vi "Test Get Test Name.vi"(8 "error in (no error)":errorcluster, 11 "Test Case In":refnum<class "Test Case Test.lvclass">) -> (0 "error out":errorcluster, 3 "Test Case Out":refnum<class "Test Case Test.lvclass">)   [LabVIEW 2020, in "Test Case Test.lvclass"]
uses:
  Test Case Test.lvclass
  C:/Program Files (x86)/National Instruments/LabVIEW 2020/vi.lib/Astemes/LUnit/Test Case.lvclass
  Test Doubles/Light Test Case Double Copy/Light Test Case Double Copy.lvclass
  C:/git/astemes-lunit/source/Core/LUnit Test Case/LUnit Test Case.lvclass
  source/LUnit Test Case.lvclass/LUnit Test Case.ctl
  <vilib>/Astemes/LUnit/Test Case.lvclass/Test Case.ctl
  e8c5eeff-a694-4c0d-b261-74e2e6f5327d.vi
  <vilib>/Astemes/LUnit/Core/LUnit Test Case/Private/Append Pass Result.vi
  <vilib>/Astemes/LUnit/Core/LUnit Test Case/Private/Append Fail Result.vi
  e8c5eeff-a694-4c0d-b261-74e2e6f5327d.vi/9c5d11cd-9439-4240-a1ee-d9baace9c924.vi
  <vilib>/Astemes/LUnit/Core/LUnit Test Case/Private/Run In UI.vi
  <vilib>/Utility/error.llb/Clear Errors.vi
  <vilib>/Utility/LVClass/Get LV Class Name.vi
  source/LUnit Test Case.lvclass
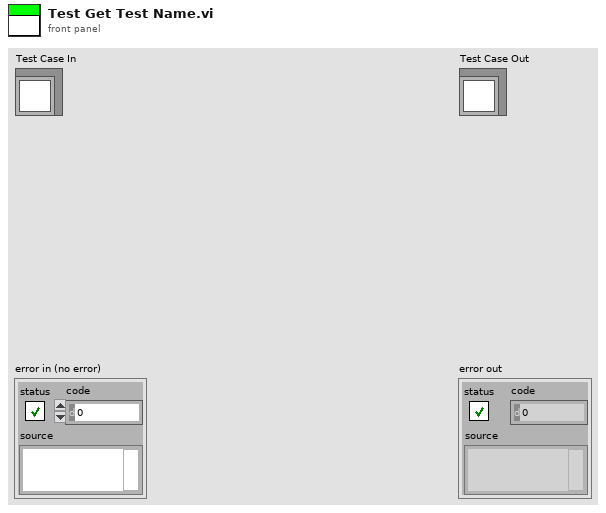
[diagram p1: front panel]
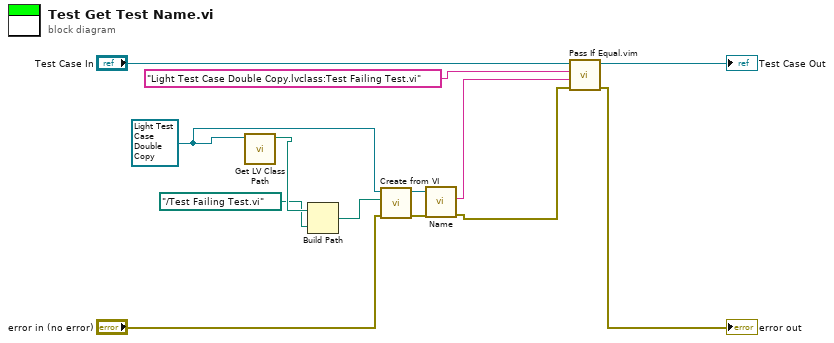
[diagram p0: block diagram]
diagram:
  w2 = refnum<class "Light Test Case Double Copy.lvclass"> refnum ("Light Test Case Double Copy.lvclass")
  n1 = call <vilib>:"Get LV Class Path.vi"("object"=w2) -> ("class path"=w10:path)  [unwired: 9 in, 1 out]
  n2 = Build Path(base path=w10, name or relative path=path "../Test Failing Test.vi" ("Relative Path from 1 to 2")) -> (appended path=w1:path)
  n3 = call "Create from VI.vi"("error in (no error)"="error in (no error)", "Test Method VI Path"=w1, "LUnit Test Case In"=w2) -> ("error out"=w7:errorcluster, "LUnit Test Case Out"=w8:refnum<class "Light Test Case Double Copy.lvclass">)  [unwired: 7 in]
  n4 = call-dynamic "Name.vi"("error in (no error)"=w7, "LUnit Test Case in"=w8) -> ("error out"=w4:errorcluster, "Name"=w6:string)  [unwired: 7 in, 1 out]
  n5 = call "Pass If Equal.vim"("error in (no error)"=w4, "Actual"=w6, "Expected"="Light Test Case Double Copy.lvclass:Test Failing Test.vi" ("Name"), "LUnit Test Case In"="Test Case In") -> ("error out"=→"error out":errorcluster, "LUnit Test Case Out"=→"Test Case Out":refnum<class "Test Case Test.lvclass">)  [unwired: 6 in]
